vi "3-5.vi"(1 "x":dbl) -> (0 "y":dbl)   [LabVIEW 2017]
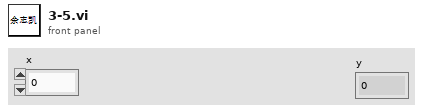
[diagram p1: front panel]
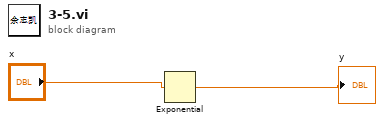
[diagram p0: block diagram]
diagram:
  n1 = Exponential(1:"x") -> (0:→"y":dbl)
